vi "Save-sequences.vi"(8 "error in (no error)":errorcluster, 11 "Available motors in":refnum<class "Motor-assembly.lvclass">) -> (0 "error out":errorcluster, 3 "Available motors out":refnum<class "Motor-assembly.lvclass">)   [LabVIEW 2013, in "PowderDeposition.lvlib" / "Motor-assembly.lvclass"]
uses:
  Motor-assembly.lvclass
  Motor-assembly.lvclass/Motor-assembly.ctl
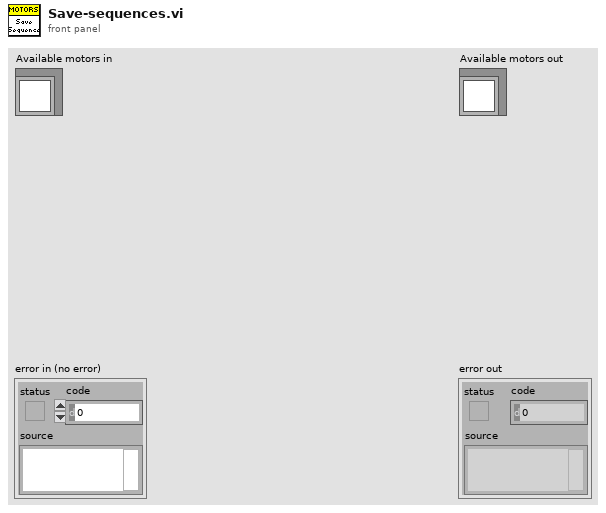
[diagram p1: front panel]
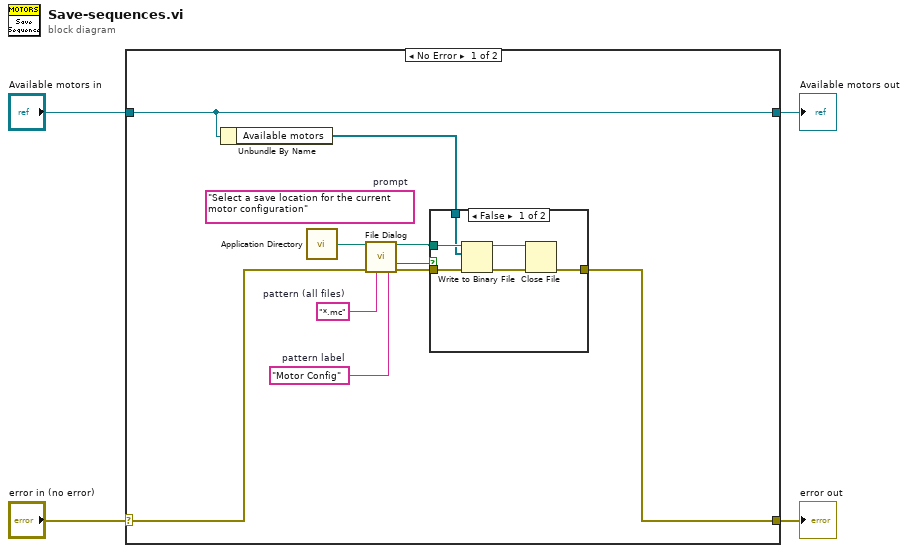
[diagram p0: block diagram]
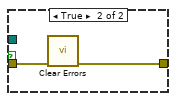
[diagram p2: hidden frame]
diagram:
  n1 = case shown="No Error" "error in (no error)" {
    selector: "error in (no error)" -> [w9 w24]
    tunnel: [w13 w24] -> w3
    tunnel: [w11 w23] -> w1
    tunnel: "Available motors in" -> [w11 w23]
    frame No Error {
      w5 = "Motor Config"  # pattern label
      w6 = "*.mc"  # pattern (all files)
      (unwired) "Select a save location for the current motor configuration"  # prompt
      n2 = Unbundle By Name(w11) -> ("Available motors"=w12:refnum<class "Motor.lvclass">[])
      n3 = call <vilib>:"Application Directory.vi"() -> ("Application Directory"=w10:path)
      n4 = call "File Dialog"("start path"=w10, "error in"=w9, "pattern (all files)"=w6, "pattern label"=w5) -> ("selected path"=w14:path, "cancelled"=w7:bool, "error out"=w8:errorcluster)  [unwired: 8 in, 1 out]
      n5 = case shown="False" w7 {
        tunnel: w8 -> [w20 w22]
        tunnel: w14 -> [w19 _]
        tunnel: [w16 w21] -> w13
        tunnel: w12 -> [w15 _]
        frame False {
          n6 = Write to Binary File(file (use dialog)=w19, data=w15, error in=w20) -> (refnum out=w17:refnum<file>, error out=w18:errorcluster)  [unwired: 3 in, 1 out]
          n7 = Close File(refnum=w17, error in=w18) -> (error out=w16:errorcluster)  [unwired: 1 out]
        }
        frame True {
          n8 = call <vilib>:"Clear Errors.vi"("error in (no error)"=w22) -> ("error out"=w21:errorcluster)  [unwired: 6 in]
        }
      }
    }
    frame Error {
    }
  }
  "error out" <- w3
  "Available motors out" <- w1
